vi "fetchChannelList.vi"(8 "error in":errorcluster, 10 "DAQ ID #":i32, 11 "Channels":string) -> (0 "error out":errorcluster, 2 "Channel Match?":bool, 3 "Read Channels":string)   [LabVIEW 2024]
uses:
  <vilib>/Utility/error.llb/Trim Whitespace One-Sided.vi
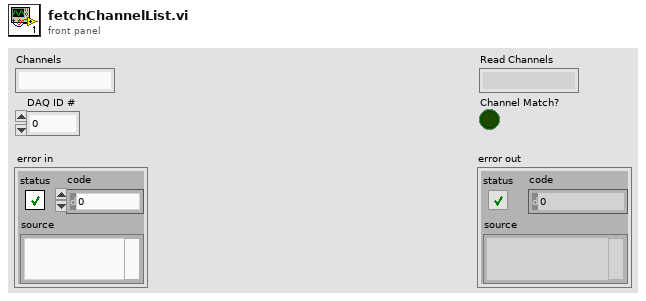
[diagram p1: front panel]
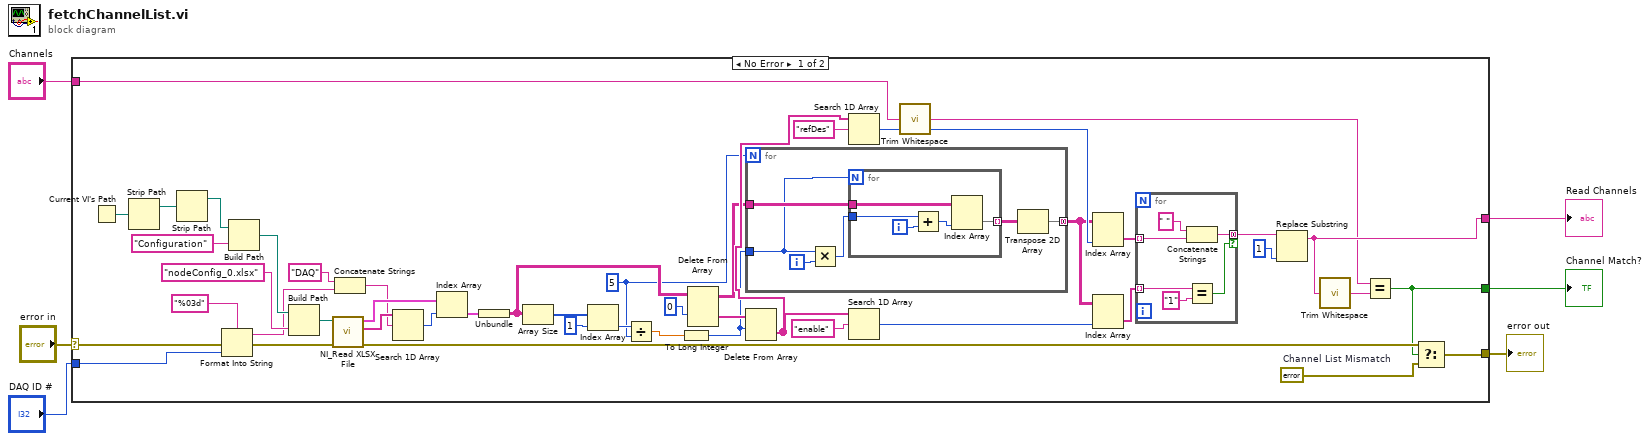
[diagram p0: block diagram]
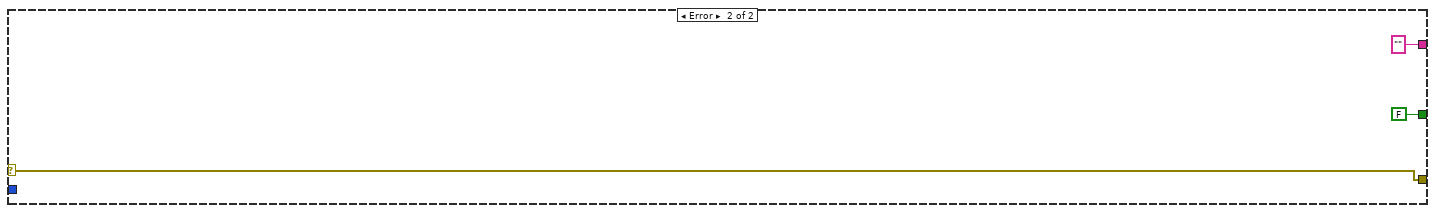
[diagram p2: hidden frame]
diagram:
  n1 = case shown="No Error" "error in" {
    selector: "error in" -> [w30 w70]
    tunnel: "DAQ ID #" -> [w36 _]
    tunnel: [w14 ""] -> w5
    tunnel: "Channels" -> [w11 _]
    tunnel: [w7 FALSE] -> w3
    tunnel: [w8 w70] -> w1
    frame No Error {
      w10 = errorcluster {"status"=TRUE, "code"=0, "source"="Channel List Mismatch"}  # Channel List Mismatch
      w23 = 5 ("y")
      n2 = Current VI's Path() -> (path=w50:path)
      n3 = Strip Path(path=w50) -> (stripped path=w47:path)  [unwired: 1 out]
      n4 = Strip Path(path=w47) -> (stripped path=w46:path)  [unwired: 1 out]
      n5 = Format Into String(format string="%03d", error in=w30, w36) -> (resulting string=w40:string, error out=w38:errorcluster)  [unwired: 1 in]
      n6 = Build Path(base path=w46, name or relative path="Configuration") -> (appended path=w48:path)
      n7 = Build Path(base path=w48, name or relative path="nodeConfig_0.xlsx") -> (appended path=w51:path)
      n8 = call "NI_Read XLSX File.vi"("error in"=w38, "XLSX File"=w51) -> ("error out"=w9:errorcluster, "Sheet Names"=w43:string[], "Sheet Data"=w45:cluster{"Array":string[][]}[])  [unwired: 7 in]
      n9 = Concatenate Strings("DAQ" ("string"), w40) -> (w42:string)
      n10 = Search 1D Array(1D array=w43, element=w42) -> (index of element=w37:i32)  [unwired: 1 in]
      n11 = Index Array(array=w45, index=w37) -> (element=w44:cluster{"Array":string[][]})
      n12 = Unbundle(w44) -> ("Array"=w29:string[][])
      n13 = Array Size(array=w29) -> (size(s)=w35:i32[])
      n14 = Index Array(array=w35, index=1) -> (element=w33:i32)
      n15 = Divide(x=w33, y=w23) -> (x/y=w31:dbl)
      n16 = To Long Integer(number=w31) -> (32bit integer=w22:i32)
      n17 = Delete From Array(array=w29, index (row)=0) -> (deleted portion=w25:string[], array with subset deleted=w24:string[][])  [unwired: 2 in]
      n18 = for {
        N: w23 -> [_]
        tunnel: w24 -> [w64]
        tunnel: w22 -> [w62]
        tunnel: [w59] -> w20 mode=concatenating
        i -> [w63]
        n19 = Multiply(x=w62, y=w63) -> (x*y=w61:i32)
        n20 = for {
          N: w62 -> [_]
          tunnel: w64 -> [w69]
          tunnel: w61 -> [w67]
          tunnel: [w65] -> w60 mode=indexing
          i -> [w68]
          n21 = Add(x=w67, y=w68) -> (x+y=w66:i32)
          n22 = Index Array(array=w69, index (col)=w66) -> (element=w65:string[])  [unwired: 1 in]
        }
        n23 = Transpose 2D Array(2D array=w60) -> (transposed array=w59:string[][])
      }
      n24 = Delete From Array(array=w25, length=w22) -> (deleted portion=w28:string[])  [unwired: 1 in, 1 out]
      n25 = Search 1D Array(1D array=w28, element="refDes") -> (index of element=w21:i32)  [unwired: 1 in]
      n26 = Search 1D Array(1D array=w28, element="enable") -> (index of element=w19:i32)  [unwired: 1 in]
      n27 = call <vilib>:"Trim Whitespace.vi"("string"=w11) -> ("trimmed string"=w12:string)  [unwired: 1 in]
      n28 = Index Array(array=w20, index (col)=w21) -> (element=w18:string[])  [unwired: 1 in]
      n29 = Index Array(array=w20, index (col)=w19) -> (element=w17:string[])  [unwired: 1 in]
      n30 = for {
        tunnel: w18 -> [w58] mode=indexing
        tunnel: w17 -> [w55] mode=indexing
        tunnel: [w57] -> w16 mode=concatenating if=w53
        n31 = Concatenate Strings(" " ("string"), w58) -> (w57:string)
        n32 = Equal?(x=w55, y="1") -> (x = y?=w53:bool)
      }
      n33 = Replace Substring(2:1 ("length (len. of substring)"), 5:w16) -> (1:w14:string)  [unwired: 2 in, 1 out]
      n34 = call <vilib>:"Trim Whitespace.vi"("string"=w14) -> ("trimmed string"=w13:string)  [unwired: 1 in]
      n35 = Equal?(x=w12, y=w13) -> (x = y?=w7:bool)
      n36 = Select(t=w9, s=w7, f=w10) -> (s? t:f=w8:errorcluster)
    }
    frame Error {
    }
  }
  "error out" <- w1
  "Read Channels" <- w5
  "Channel Match?" <- w3
